vi "PID (generic).vi"(6 "reinitialize? (F)":bool, 7 "output range (-1, 1)":cluster{"output high":dbl, "output low":dbl}={"output high"=1.0, "output low"=-1.0}, 9 "PID gains":T2={"proportional gain (Kc)"=0.05, "integral time (Ti, min)"=0.003, "derivative time (Td, min)"=0.0} {"derivative time (Td, min)" format="%.6f"; "integral time (Ti, min)" format="%.6f"; "proportional gain (Kc)" format="%.6f"}, 10 "dx/dt (measured)":dbl, 11 "Setpoint":dbl(slide)=-0.016713091922005565 scale=-2.0..2.0) -> (0 "dt out (s)":dbl format="%.3f", 1 "dx/dt":dbl, 2 "output":dbl format="%.2f", 3 "Speed Graph":T1(graph))   [LabVIEW 2017]
uses:
  <vilib>/addons/control/pid/pid.llb/PID (DBL).vi
  <vilib>/addons/control/pid/NI_PID_pid.lvlib
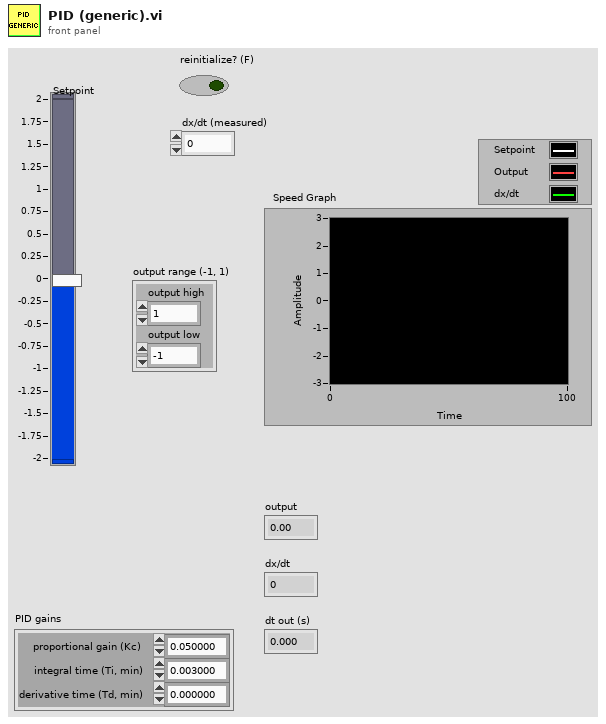
[diagram p1: front panel]
types:
  T1 = cluster{"Setpoint":dbl, "output":dbl, "dx/dt":dbl}
  T2 = cluster{"proportional gain (Kc)":dbl, "integral time (Ti, min)":dbl, "derivative time (Td, min)":dbl}
  T3 = cluster{"Setpoint":dbl, "output":dbl, "dx/dt (measured)":dbl}
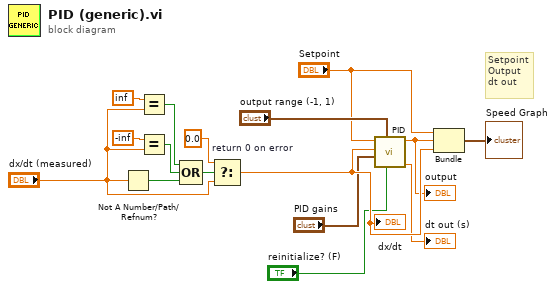
[diagram p0: block diagram]
diagram:
  # "Setpoint\nOutput\ndt out"
  n1 = Not A Number/Path/Refnum?(number/path/refnum="dx/dt (measured)") -> (NaN/Path/Refnum?=w3:bool)
  n2 = Equal?(x=inf, y="dx/dt (measured)") -> (x = y?=w7:bool)
  n3 = Equal?(x=-inf, y="dx/dt (measured)") -> (x = y?=w4:bool)
  n4 = Compound Arithmetic op=OR(w7, w4, w3) -> (w2:bool)
  n5 = Select "return 0 on error"(t=0.0, s=w2, f="dx/dt (measured)") -> (s? t:f=w16:dbl)
  "dx/dt" <- w16
  n6 = call-poly <vilib>:"PID.vi"("reinitialize? (F)"="reinitialize? (F)", "output range"="output range (-1, 1)", "PID gains"="PID gains", "process variable"=w16, "setpoint"="Setpoint") -> ("dt out (s)"=→"dt out (s)":dbl, "output"=w13:dbl)  [unwired: 5 in]
  "output" <- w13
  n7 = Bundle("Setpoint"="Setpoint", "output"=w13, "dx/dt (measured)"=w16) -> (→"Speed Graph":T3)  [unwired: 1 in]
